vi "Find.vi"(8 "error in (no error)":errorcluster, 10 "Name":string, 11 "World In":refnum<class "3D Object.lvclass">) -> (0 "error out":errorcluster, 2 "Object out":refnum<class "3D Object.lvclass">, 3 "World Out":refnum<class "3D Object.lvclass">)   [LabVIEW 2015, in "3D Object.lvclass"]
uses:
  3D Object.lvclass
  3D Object.lvclass/3D Object.ctl
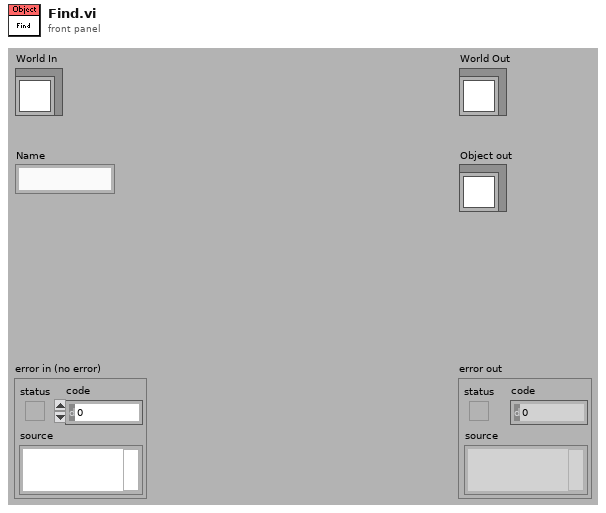
[diagram p1: front panel]
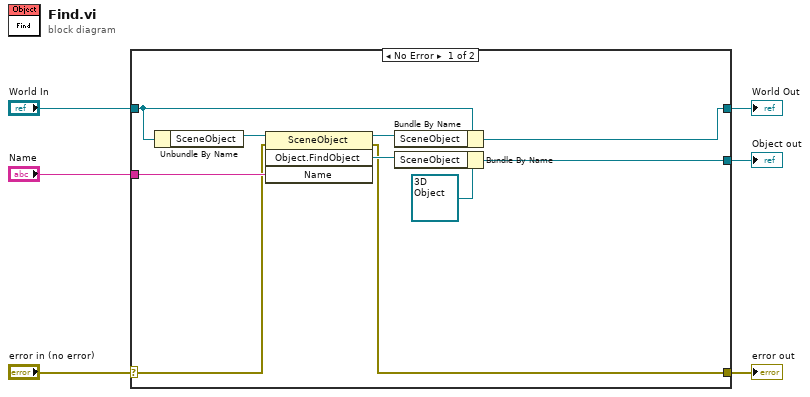
[diagram p0: block diagram]
diagram:
  n1 = case shown="No Error" "error in (no error)" {
    selector: "error in (no error)" -> [w9 w18]
    tunnel: [w8 w18] -> w5
    tunnel: [w10 w17] -> w3
    tunnel: "World In" -> [w11 w17]
    tunnel: "Name" -> [w15 _]
    tunnel: [w7 _] -> w1
    frame No Error {
      n2 = Unbundle By Name(w11) -> ("SceneObject"=w16:refnum<vi>)
      n3 = invoke class="SceneObject" method="Object.FindObject"(reference=w16, error in=w9, "Name"=w15) -> (reference out=w12:refnum<vi>, error out=w8:errorcluster, "FindObject"=w13:refnum<vi>)  [unwired: 1 in, 1 out]
      n4 = Bundle By Name(cluster=w11, "SceneObject"=w12) -> (w10:refnum<class "3D Object.lvclass">)
      n5 = Bundle By Name(cluster=refnum<class "3D Object.lvclass"> refnum ("3D Object.lvclass"), "SceneObject"=w13) -> (w7:refnum<class "3D Object.lvclass">)
    }
    frame Error {
    }
  }
  "error out" <- w5
  "World Out" <- w3
  "Object out" <- w1
